vi "Subvi_IntakeLiftPosition_Teleop.vi"(11 "setpoint":dbl) -> (2 "voltage out":dbl, 3 "Cluster":cluster{"setpoint":dbl, "Distance":dbl})   [LabVIEW 2017]
doc: "this VI takes a target and makes the intake lift go to said target"
uses:
  <vilib>/addons/control/pid/pid.llb/PID (DBL).vi
  <vilib>/addons/control/pid/NI_PID_pid.lvlib
panel:
  out "Target/actual":cluster{dbl, "Distance":dbl}(graph)
  out "voltage/output":dbl(graph)
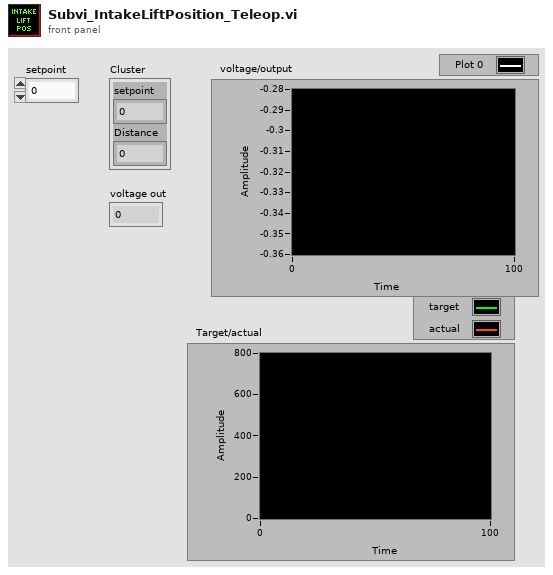
[diagram p1: front panel]
types:
  T1 = cluster{"proportional gain (Kc)":dbl, "integral time (Ti, min)":dbl, "derivative time (Td, min)":dbl}
  T2 = typedef "WPI_EncoderDevRef.ctl" = cluster{"DevStatus":errorcluster, "EncoderIndex":T3, "CounterIndex":T4, "DistancePerCount":dbl, "Decoding Type":T5}
  T3 = typedef "FPGA_EncoderIdx.ctl" = enum8{"Enc 0", "Enc 1", "Enc 2", "Enc 3", "Enc 4", "Enc 5", "Enc 6", "Enc 7", "Invalid"}
  T4 = typedef "FPGA_CounterCtrSystemIndex.ctl" = enum8{"Ctr 0", "Ctr 1", "Ctr 2", "Ctr 3", "Ctr 4", "Ctr 5", "Ctr 6", "Ctr 7", "Invalid"}
  T5 = typedef "WPI_EncoderType.ctl" = enum16{"1x", "2x", "4x"}
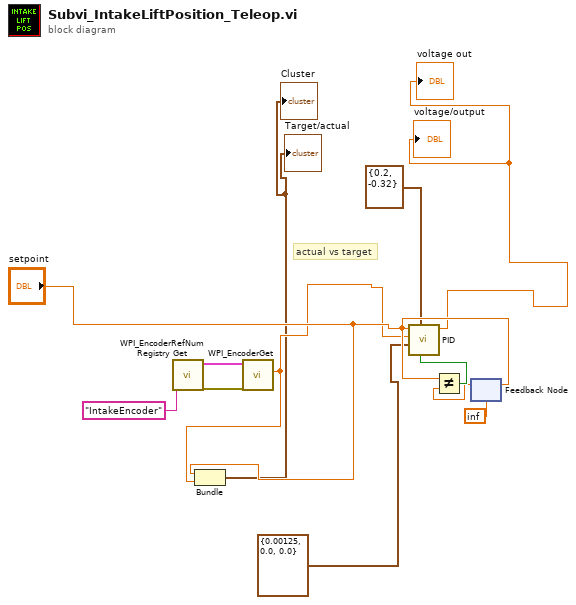
[diagram p0: block diagram]
diagram:
  # "actual vs target"
  n1 = call <vilib>:"WPI_EncoderRefNum Registry Get.vi"("refnum name"="IntakeEncoder") -> ("error out"=w4:errorcluster, "EncoderDevRef"=w3:T2)  [unwired: 9 in]
  n2 = call <vilib>:"WPI_EncoderGet.vi"("error in (no error)"=w4, "EncoderDevRef"=w3) -> ("Distance"=w8:dbl)  [unwired: 4 in, 5 out]
  n3 = Bundle("setpoint"="setpoint", "Distance"=w8) -> (→"Cluster" →"Target/actual":cluster{"setpoint":dbl, "Distance":dbl})  [unwired: 1 in]
  n4 = feedback #1(inf ("setpoint")) -> (w10:dbl)
  n5 = Not Equal?(x="setpoint", y=w10) -> (x != y?=w11:bool)
  n6 = call-poly <vilib>:"PID.vi"("reinitialize? (F)"=w11, "output range"=cluster{"output high":dbl, "output low":dbl} {"output high"=0.2, "output low"=-0.32}, "PID gains"=T1 {"proportional gain (Kc)"=0.00125, "integral time (Ti, min)"=0.0, "derivative time (Td, min)"=0.0}, "process variable"=w8, "setpoint"="setpoint") -> ("output"=→"voltage out" →"voltage/output":dbl)  [unwired: 5 in, 1 out]
  n7 = feedback-in #1("setpoint") -> ()
